vi "Host_RunVI.vi"(11 "VI in":refnum<vi>) -> ()   [LabVIEW 2018]
doc: "Runs the vi of the input reference and opens the front panel.\nIf the function is called while the vi is already running, the vi will instead be aborted and closed."
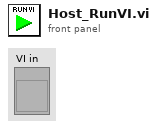
[diagram p1: front panel]
types:
  T1 = enum32{"Bad", "Idle", "Run top level", "Running"}
  T2 = enum32{"Invalid", "Standard", "Closed", "Hidden", "Minimized", "Maximized"}
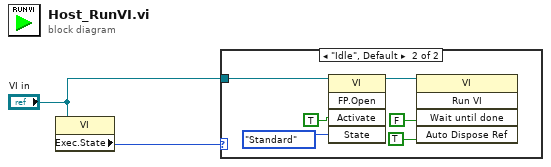
[diagram p0: block diagram]
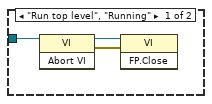
[diagram p2: hidden frame]
diagram:
  n1 = property class="VI"(reference="VI in") -> ("Exec.State"=w2:T1)  [unwired: 1 in, 2 out]
  n2 = case shown="\"Idle\", Default" w2 {
    tunnel: "VI in" -> [w5 w6]
    frame "Run top level", "Running" {
      n3 = invoke class="VI" method="Abort VI"(reference=w5) -> (reference out=w4:refnum<vi>, error out=w3:errorcluster)  [unwired: 2 in, 1 out]
      n4 = invoke class="VI" method="FP.Close"(reference=w4, error in=w3) -> ()  [unwired: 1 in, 3 out]
    }
    frame "Idle", Default {
      n5 = invoke class="VI" method="FP.Open"(reference=w6, "Activate"=TRUE ("Activate?"), "State"=T2."Standard") -> (reference out=w9:refnum<vi>)  [unwired: 2 in, 4 out]
      n6 = invoke class="VI" method="Run VI"(reference=w9, "Wait until done"=FALSE ("Wait Until Done"), "Auto Dispose Ref"=TRUE ("Auto Dispose Reference")) -> ()  [unwired: 2 in, 5 out]
    }
  }
